vi "RPC Open Driver App Reference.vi"(7 "port number (3363)":u16=3363, 8 "error in (no error)":errorcluster, 9 "Driver ID (\"\")":string, 10 "Driver Type (\"\")":string, 11 "Client (\"\": open server reference)":string) -> (0 "error out":errorcluster, 1 "Driver Config Path":path, 2 "Driver Component Path":path, 3 "app reference":refnum<vi>)   [LabVIEW 2011]
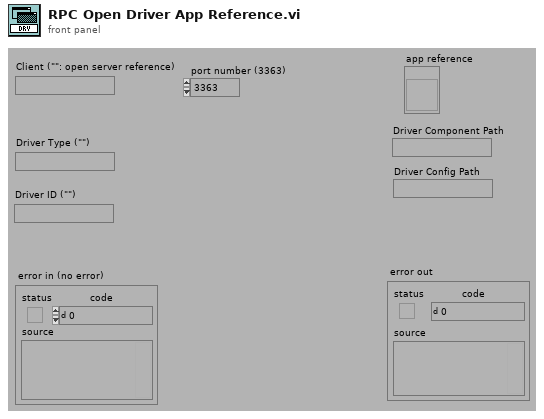
[diagram p1: front panel]
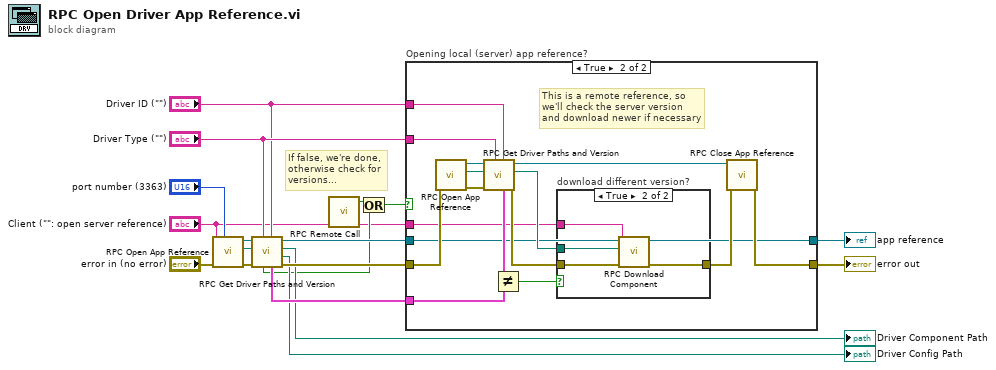
[diagram p0: block diagram]
diagram:
  # "If false, we're done,\notherwise check for\nversions..."
  n1 = call "RPC Open App Reference.vi"("Port Number (3363)"="port number (3363)", "error in (no error)"="error in (no error)", "Client (\"\": open server reference)"="Client (\"\": open server reference)") -> ("error out"=w12:errorcluster, "Component Base Path"=w9:path, "App Reference"=w14:refnum<vi>)  [unwired: 2 in, 4 out]
  n2 = call "RPC Get Driver Paths and Version.vi"("Driver ID (\"\")"="Driver ID (\"\")", "Driver Type (\"\")"="Driver Type (\"\")", "error in (no error)"=w12, "Base Path (empty)"=w9, "app reference (empty)"=w14) -> ("error out"=w11:errorcluster, "Driver Config Path"=→"Driver Config Path":path, "Driver Component Path"=→"Driver Component Path":path, "app reference"=w13:refnum<vi>, "Component Version"=w10:cluster{"Version":string, "Build Number":u32}, "version error?"=w3:bool)  [unwired: 1 in]
  n3 = call "RPC Remote Call.vi"("IP (\"\")"="Client (\"\": open server reference)") -> ("Remote Call?"=w1:bool)  [unwired: 4 out]
  n4 = Or(x=w1, y=w3) -> (x .or. y?=w4:bool)
  n5 = case "Opening local (server) app reference?" shown="True" w4 {
    tunnel: w11 -> [w19 w36]
    tunnel: w13 -> [w20 w22]
    tunnel: [w20 w22] -> w17
    tunnel: [w19 w33] -> w16
    tunnel: "Driver Type (\"\")" -> [_ w28]
    tunnel: "Driver ID (\"\")" -> [_ w27]
    tunnel: w10 -> [_ w32]
    tunnel: "Client (\"\": open server reference)" -> [_ w21]
    frame False {
    }
    frame True {
      # "This is a remote reference, so\nwe'll check the server version\nand download newer if necessary"
      n6 = call "RPC Open App Reference.vi"("error in (no error)"=w36) -> ("error out"=w25:errorcluster, "Component Base Path"=w29:path, "App Reference"=w31:refnum<vi>)  [unwired: 4 in, 4 out]
      n7 = call "RPC Get Driver Paths and Version.vi"("Driver ID (\"\")"=w27, "Driver Type (\"\")"=w28, "error in (no error)"=w25, "Base Path (empty)"=w29, "app reference (empty)"=w31) -> ("error out"=w24:errorcluster, "Driver Component Path"=w23:path, "app reference"=w30:refnum<vi>, "Component Version"=w26:cluster{"Version":string, "Build Number":u32})  [unwired: 3 out]
      n8 = Not Equal?(x=w26, y=w32) -> (x != y?=w35:bool)
      n9 = case "download different version?" shown="True" w35 {
        tunnel: w24 -> [w37 w41]
        tunnel: [w37 w40] -> w34
        tunnel: w23 -> [_ w38]
        tunnel: w21 -> [_ w39]
        frame False {
        }
        frame True {
          n10 = call "RPC Download Component.vi"("error in (no error)"=w41, "Component Path (empty)"=w38, "Client (\"\")"=w39) -> ("error out"=w40:errorcluster)  [unwired: 8 out]
        }
      }
      n11 = call "RPC Close App Reference.vi"("error in (no error)"=w34, "app reference"=w30) -> ("error out"=w33:errorcluster)  [unwired: 9 out]
    }
  }
  "error out" <- w16
  "app reference" <- w17
